vi "RabiMeasurement_IQ2.vi"() -> ()   [LabVIEW 2020]
uses:
  <vilib>/Swabian Instruments/Pulse Streamer/PulseStreamer/PulseStreamer/typedefs/typedef_TriggerStart.ctl
  Host Subvi's/Control 3.ctl
  <vilib>/Swabian Instruments/Pulse Streamer/PulseStreamer/typedefs/typedef_OutputState.ctl
  <vilib>/Swabian Instruments/Pulse Streamer/PulseStreamer/typedefs/typedef_ChannelNumber.ctl
  <vilib>/Swabian Instruments/Pulse Streamer/PulseStreamer/PulsePattern/PulsePattern.lvclass
  C:/Program Files (x86)/National Instruments/LabVIEW 2020/vi.lib/Swabian Instruments/Pulse Streamer/PulseStreamer/Pattern/Pattern.lvclass
  <vilib>/Swabian Instruments/Pulse Streamer/PulseStreamer/Sequence/Sequence.lvclass/Sequence.ctl
  <vilib>/Swabian Instruments/Pulse Streamer/PulseStreamer/AnalogPattern/AnalogPattern.lvclass
  <vilib>/FPGAPlugInAG/USB-7855R/niLvFpga_Open_USB-7855R.vi
  <vilib>/rvi/interface/common/dynamic/niFpgaDynamicAddResources.vi
  <vilib>/rvi/interface/common/niFpgaWaitOnOcc.vi
  <vilib>/Utility/error.llb/Error Cluster From Error Code.vi
  <vilib>/rvi/errors/niLvFpgaAdjustHostInterfaceError.vi
  <vilib>/Swabian Instruments/Pulse Streamer/PulseStreamer/Pattern/Read total duration.vi
  <vilib>/Swabian Instruments/Pulse Streamer/PulseStreamer/PulseStreamer/stream/stream (Sequence).vi
  <vilib>/FPGAPlugInAG/Dynamic/niLvFpga_Close_Dynamic.vi
  <vilib>/rvi/interface/nirviOpenFPGA/nirviOpenFPGA.xnode
  FPGA Bitfiles/EverythingDAQ_FPGATarget2_FPGARabiver2_krdpsiHB5ks.lvbitx
  FPGA_Readout.vi
  <vilib>/rvi/interface/nirviMethod/nirviMethod.xnode
  <vilib>/rvi/interface/nirviCloseFPGA/nirviCloseFPGA.xnode
  <vilib>/Swabian Instruments/Pulse Streamer/PulseStreamer/PulseStreamer/PulseStreamer.lvclass
  <vilib>/Swabian Instruments/Pulse Streamer/PulseStreamer/Sequence/Sequence.lvclass
  <vilib>/FPGAPlugInAG/Dynamic/niLvFpga_ConfigureFifo_Dynamic.vi
  <vilib>/rvi/errors/niLvFpgaMergeErrorWithErrorCode.vi
  <vilib>/FPGAPlugInAG/Dynamic/niLvFpga_WriteFifo_Dynamic.vi
  <vilib>/FPGAPlugInAG/Dynamic/niLvFpga_ReadFifo_Dynamic.vi
  <vilib>/Swabian Instruments/Pulse Streamer/PulseStreamer/PulseStreamer.lvlib
panel:
  out "ESR F2":cluster{"tau array":dbl[], dbl[]}(graph)
  out "ESR F1":cluster{"tau array":dbl[], dbl[]}(graph)
  out "Ave F2":dbl[](array[numeric]) format="%.2f"
  out "Ave F1":dbl[](array[numeric]) format="%.2f"
  out "64bit integer":dbl=22.88
  out "tau array":dbl[](array[numeric])=[2.5, 5.0, 7.5, 10.0, 12.5, 15.0, 17.5, 20.0, 22.5, 25.0, 27.5, 30.0, 32.5, 35.0, 37.5, 40.0, 42.5, 45.0, 47.5, 50.0, 52.5, 55.0, 57.5, 60.0, 62.5, 65.0, 67.5, 70.0, 72.5, 75.0, 77.5, 80.0, 82.5, 85.0, 87.5, 90.0, 92.5, 95.0, 97.5, 100.0, 102.5, 105.0, 107.5, 110.0, 112.5, 115.0, 117.5, 120.0, 122.5, 125.0, 127.5, 130.0, 132.5, 135.0, 137.5, 140.0, 142.5, 145.0, 147.5, 150.0, 152.5, 155.0, 157.5, 160.0, 162.5, 165.0, 167.5, 170.0, 172.5, 175.0, 177.5, 180.0, 182.5, 185.0, 187.5, 190.0, 192.5, 195.0, 197.5, 200.0, 202.5, 205.0, 207.5, 210.0, 212.5, 215.0, 217.5, 220.0, 222.5, 225.0, 227.5, 230.0, 232.5, 235.0, 237.5, 240.0, 242.5, 245.0, 247.5, 250.0, 252.5, 255.0, 257.5, 260.0, 262.5, 265.0, 267.5, 270.0, 272.5, 275.0, 277.5, 280.0, 282.5, 285.0, 287.5, 290.0, 292.5, 295.0, 297.5, 300.0, 302.5, 305.0, 307.5, 310.0, 312.5, 315.0, 317.5, 320.0, 322.5, 325.0, 327.5, 330.0, 332.5, 335.0, 337.5, 340.0, 342.5, 345.0, 347.5, 350.0, 352.5, 355.0, 357.5, 360.0, 362.5, 365.0, 367.5, 370.0, 372.5, 375.0, 377.5, 380.0, 382.5, 385.0, 387.5, 390.0, 392.5, 395.0, 397.5, 400.0, 402.5, 405.0, 407.5, 410.0, 412.5, 415.0, 417.5, 420.0, 422.5, 425.0, 427.5, 430.0, 432.5, 435.0, 437.5, 440.0, 442.5, 445.0, 447.5, 450.0, 452.5, 455.0, 457.5, 460.0, 462.5, 465.0, 467.5, 470.0, 472.5, 475.0, 477.5, 480.0, 482.5, 485.0, 487.5, 490.0, 492.5, 495.0, 497.5, 500.0, 502.5, 505.0, 507.5, 510.0, 512.5, 515.0, 517.5, 520.0, 522.5, 525.0, 527.5, 530.0, 532.5, 535.0, 537.5, 540.0, 542.5, 545.0, 547.5, 550.0, 552.5, 555.0, 557.5, 560.0, 562.5, 565.0, 567.5, 570.0, 572.5, 575.0, 577.5, 580.0, 582.5, 585.0, 587.5, 590.0, 592.5, 595.0, 597.5, 600.0, 602.5, 605.0, 607.5, 610.0, 612.5, 615.0, 617.5, 620.0, 622.5, 625.0, 627.5, 630.0, 632.5, 635.0, 637.5, 640.0, 642.5, 645.0, 647.5, 650.0, 652.5, 655.0, 657.5, 660.0, 662.5, 665.0, 667.5, 670.0, 672.5, 675.0, 677.5, 680.0, 682.5, 685.0, 687.5, 690.0, 692.5, 695.0, 697.5, 700.0, 702.5, 705.0, 707.5, 710.0, 712.5, 715.0, 717.5, 720.0, 722.5, 725.0, 727.5, 730.0, 732.5, 735.0, 737.5, 740.0, 742.5, 745.0, 747.5, 750.0, 752.5, 755.0, 757.5, 760.0, 762.5, 765.0, 767.5, 770.0, 772.5, 775.0, 777.5, 780.0, 782.5, 785.0, 787.5, 790.0, 792.5, 795.0, 797.5, 800.0, 802.5, 805.0, 807.5, 810.0, 812.5, 815.0, 817.5, 820.0, 822.5, 825.0, 827.5, 830.0, 832.5, 835.0, 837.5, 840.0, 842.5, 845.0, 847.5, 850.0, 852.5, 855.0, 857.5, 860.0, 862.5, 865.0, 867.5, 870.0, 872.5, 875.0, 877.5, 880.0, 882.5, 885.0, 887.5, 890.0, 892.5, 895.0, 897.5, 900.0, 902.5, 905.0, 907.5, 910.0, 912.5, 915.0, 917.5, 920.0, 922.5, 925.0, 927.5, 930.0, 932.5, 935.0, 937.5, 940.0, 942.5, 945.0, 947.5, 950.0, 952.5, 955.0, 957.5, 960.0, 962.5, 965.0, 967.5, 970.0, 972.5, 975.0, 977.5, 980.0, 982.5, 985.0, 987.5, 990.0, 992.5, 995.0, 997.5, 1000.0, 1002.5, 1005.0, 1007.5, 1010.0, 1012.5, 1015.0, 1017.5, 1020.0, 1022.5, 1025.0, 1027.5, 1030.0, 1032.5, 1035.0, 1037.5, 1040.0, 1042.5, 1045.0, 1047.5, 1050.0, 1052.5, 1055.0, 1057.5, 1060.0, 1062.5, 1065.0, 1067.5, 1070.0, 1072.5, 1075.0, 1077.5, 1080.0, 1082.5, 1085.0, 1087.5, 1090.0, 1092.5, 1095.0, 1097.5, 1100.0, 1102.5, 1105.0, 1107.5, 1110.0, 1112.5, 1115.0, 1117.5, 1120.0, 1122.5, 1125.0, 1127.5, 1130.0, 1132.5, 1135.0, 1137.5, 1140.0, 1142.5, 1145.0, 1147.5, 1150.0, 1152.5, 1155.0, 1157.5, 1160.0, 1162.5, 1165.0, 1167.5, 1170.0, 1172.5, 1175.0, 1177.5, 1180.0, 1182.5, 1185.0, 1187.5, 1190.0, 1192.5, 1195.0, 1197.5, 1200.0, 1202.5, 1205.0, 1207.5, 1210.0, 1212.5, 1215.0, 1217.5, 1220.0, 1222.5, 1225.0, 1227.5, 1230.0, 1232.5, 1235.0, 1237.5, 1240.0, 1242.5, 1245.0, 1247.5, 1250.0, 1252.5, 1255.0, 1257.5, 1260.0, 1262.5, 1265.0, 1267.5, 1270.0, 1272.5, 1275.0, 1277.5, 1280.0, 1282.5, 1285.0, 1287.5, 1290.0, 1292.5, 1295.0, 1297.5, 1300.0, 1302.5, 1305.0, 1307.5, 1310.0, 1312.5, 1315.0, 1317.5, 1320.0, 1322.5, 1325.0, 1327.5, 1330.0, 1332.5, 1335.0, 1337.5, 1340.0, 1342.5, 1345.0, 1347.5, 1350.0, 1352.5, 1355.0, 1357.5, 1360.0, 1362.5, 1365.0, 1367.5, 1370.0, 1372.5, 1375.0, 1377.5, 1380.0, 1382.5, 1385.0, 1387.5, 1390.0, 1392.5, 1395.0, 1397.5, 1400.0, 1402.5, 1405.0, 1407.5, 1410.0, 1412.5, 1415.0, 1417.5, 1420.0, 1422.5, 1425.0, 1427.5, 1430.0, 1432.5, 1435.0, 1437.5, 1440.0, 1442.5, 1445.0, 1447.5, 1450.0, 1452.5, 1455.0, 1457.5, 1460.0, 1462.5, 1465.0, 1467.5, 1470.0, 1472.5, 1475.0, 1477.5, 1480.0, 1482.5, 1485.0, 1487.5, 1490.0, 1492.5, 1495.0, 1497.5, 1500.0, 1502.5, 1505.0, 1507.5, 1510.0, 1512.5, 1515.0, 1517.5, 1520.0, 1522.5, 1525.0, 1527.5, 1530.0, 1532.5, 1535.0, 1537.5, 1540.0, 1542.5, 1545.0, 1547.5, 1550.0, 1552.5, 1555.0, 1557.5, 1560.0, 1562.5, 1565.0, 1567.5, 1570.0, 1572.5, 1575.0, 1577.5, 1580.0, 1582.5, 1585.0, 1587.5, 1590.0, 1592.5, 1595.0, 1597.5, 1600.0, 1602.5, 1605.0, 1607.5, 1610.0, 1612.5, 1615.0, 1617.5, 1620.0, 1622.5, 1625.0, 1627.5, 1630.0, 1632.5, 1635.0, 1637.5, 1640.0, 1642.5, 1645.0, 1647.5, 1650.0, 1652.5, 1655.0, 1657.5, 1660.0, 1662.5, 1665.0, 1667.5, 1670.0, 1672.5, 1675.0, 1677.5, 1680.0, 1682.5, 1685.0, 1687.5, 1690.0, 1692.5, 1695.0, 1697.5, 1700.0, 1702.5, 1705.0, 1707.5, 1710.0, 1712.5, 1715.0, 1717.5, 1720.0, 1722.5, 1725.0, 1727.5, 1730.0, 1732.5, 1735.0, 1737.5, 1740.0, 1742.5, 1745.0, 1747.5, 1750.0, 1752.5, 1755.0, 1757.5, 1760.0, 1762.5, 1765.0, 1767.5, 1770.0, 1772.5, 1775.0, 1777.5, 1780.0, 1782.5, 1785.0, 1787.5, 1790.0, 1792.5, 1795.0, 1797.5, 1800.0, 1802.5, 1805.0, 1807.5, 1810.0, 1812.5, 1815.0, 1817.5, 1820.0, 1822.5, 1825.0, 1827.5, 1830.0, 1832.5, 1835.0, 1837.5, 1840.0, 1842.5, 1845.0, 1847.5, 1850.0, 1852.5, 1855.0, 1857.5, 1860.0, 1862.5, 1865.0, 1867.5, 1870.0, 1872.5, 1875.0, 1877.5, 1880.0, 1882.5, 1885.0, 1887.5, 1890.0, 1892.5, 1895.0, 1897.5, 1900.0, 1902.5, 1905.0, 1907.5, 1910.0, 1912.5, 1915.0, 1917.5, 1920.0, 1922.5, 1925.0, 1927.5, 1930.0, 1932.5, 1935.0, 1937.5, 1940.0, 1942.5, 1945.0, 1947.5, 1950.0, 1952.5, 1955.0, 1957.5, 1960.0, 1962.5, 1965.0, 1967.5, 1970.0, 1972.5, 1975.0, 1977.5, 1980.0, 1982.5, 1985.0, 1987.5, 1990.0, 1992.5, 1995.0, 1997.5, 2000.0]
  out "t_tot single sequence (ns)":dbl=14300.0
  out "error out 5":errorcluster
  out "Cycle Number 2":i32=70
  in  "Cycle Initialize Tab":enum32{"uWave"}(tab)
  in  "GPIB RF":string="0:27"
  in  "RF Freq (Hz)":dbl=2170000000.0 format="%.5e"
  in  "RF Power (dBm)":dbl=-6.0 format="%.2f"
  in  "uWave Enable":bool=TRUE
  out "RF Freq Set (GHz)":dbl=2.17 format="%#_10f"
  in  "Delay (ns)":T1=760
  in  "start":T2
  in  "ip":string="169.254.8.2"
  in  "?":enum32{"Confocal"}(tab)
  in  "x":i16=77
  in  "y":i16=76
  in  "Scan Area":i16=1
  in  "Scale (1-30)":i16=4
  in  "Sample per Axis":i16=151
  in  "?":enum32{"Rabi"}(tab)
  in  "Wait Time (ns)":u32=2300
  in  "Initialization time (ns)":u32=5240
  in  "Readout (ns)":u32=6000
  in  "Number of points":u32=800
  in  "Pulse Num":u32=500
  in  "Experiment Repeat":i32=500
  out "Experiment number":i32=95
  out "n_runs":i64=500
  in  "tau start (ns)":dbl=2.5
  in  "tau step (ns)":dbl=2.5
  out "error out 4":errorcluster
  out "Digital plot":cluster{"CumTime":i64[], dbl[]}[](graph)
  out "error out 3":errorcluster
  out "Sequence duration [ms]":dbl=11440.0 format="%.2f"
  out "N_array":i32[](array[numeric])=[0, 1, 2, 3, 4, 5, 6, 7, 8, 9, 10, 11, 12, 13, 14, 15, 16, 17, 18, 19, 20, 21, 22, 23, 24, 25, 26, 27, 28, 29, 30, 31, 32, 33, 34, 35, 36, 37, 38, 39, 40, 41, 42, 43, 44, 45, 46, 47, 48, 49, 50, 51, 52, 53, 54, 55, 56, 57, 58, 59, 60, 61, 62, 63, 64, 65, 66, 67, 68, 69, 70, 71, 72, 73, 74, 75, 76, 77, 78, 79, 80, 81, 82, 83, 84, 85, 86, 87, 88, 89, 90, 91, 92, 93, 94, 95]
  out "CountAverage":dbl[](array[numeric])=[2.2072775, 2.1462875, 2.1518225, 2.13079, 2.1088175, 2.0855425, 2.092535, 2.095995, 2.059395, 2.043535, 2.0711575, 2.0722175, 2.0613325, 2.0553225, 2.05686, 2.06965, 2.0412975, 2.0224125, 2.03104, 2.0491125, 2.0315925, 2.05474, 2.070495, 2.0499125, 2.00775, 2.0107775, 1.981505, 1.9941775, 1.9933125, 1.97172, 1.9845575, 1.998325, 1.9735575, 1.9803825, 2.006115, 1.999575, 2.010875, 1.9825875, 1.9527725, 1.9487225, 1.9575375, 1.94913, 1.9602425, 1.97378, 1.9248975, 1.95134, 1.95578, 1.93173, 1.96891, 1.9429025, 1.94519, 1.9535725, 1.982075, 1.9884975, 2.0101, 2.0035625, 1.9885975, 1.9950825, 1.9905625, 2.0166725, 2.0082125, 1.979385, 1.9926625, 1.99645, 1.96617, 1.994985, 2.02208, 2.02243, 1.98502, 2.030615, 1.95893, 1.950755, 1.954205, 1.9540825, 2.001115, 2.0058825, 1.98758, 2.0253575, 2.0277525, 2.018475, 2.0500375, 1.996235, 2.002115, 1.98259, 1.9926, 2.0195225, 2.03915, 2.005845, 1.9993925, 1.97835, 1.97021, 1.971995, 1.9831425, 2.0152025, 2.005475]
  out "Averaged ESR":dbl[](array[numeric])=[1.017870567091982, 1.0428926603215876, 1.0764184990280088, 1.08249192001354, 1.09429499579298, 1.1037168082128996, 1.1050716542744574, 1.1014298057989265, 1.089578613265814, 1.0709781534452711, 1.061324574848865, 1.0399698584374584, 1.0274961657701196, 1.0323259829375757, 1.049009998093537, 1.06086353915061, 1.073642946086008, 1.0916880804324838, 1.1136897270610668, 1.1028359205101759, 1.1019091471026512, 1.0875769519321419, 1.0844743820788172, 1.0759806167827617, 1.0442674590752932, 1.048090882105439, 1.0495594176031688, 1.0518328239293575, 1.0687563191014522, 1.0818212468587356, 1.0882605899283622, 1.096100309473077, 1.1037350318350123, 1.1156983902933313, 1.1020839762563372, 1.0905140527288388, 1.0815812888771692, 1.0642144974277141, 1.0579398581706974, 1.0586754609636846, 1.0624506346078841, 1.0634495683486118, 1.0700074839543063, 1.07995537502229, 1.0894526493826528, 1.1013206815502923, 1.1003407028071455, 1.1022423549057012, 1.0954878362287324, 1.088062027708647, 1.0833266346542303, 1.076664423393035, 1.078449296773364, 1.0705152899378316, 1.0706985926619503, 1.0773806630088303, 1.0862648694729151, 1.0947271213098375, 1.098040473863476, 1.1057727933875288, 1.1001579636399577, 1.100441019528767, 1.0887476609105367, 1.0937902660037309, 1.0787961808148738, 1.0767806248990635, 1.0723241131589933, 1.0745023953966337, 1.0772759452030733, 1.0802973083495904, 1.089253522438231, 1.095749559409236, 1.0918005448710129, 1.1055463304557207, 1.0999171683721327, 1.1008361418047856, 1.092833534540528, 1.0890529342944788, 1.095166497145744, 1.0889157153776328, 1.085628303208282, 1.0781862682944452, 1.0821695429125877, 1.0925768644288618, 1.098383847187047, 1.0944772252952568, 1.1023227543449177, 1.097807910096037, 1.1009879373329856, 1.0877833673466615, 1.0861943902564453, 1.0938514691759695, 1.0973681152773327, 1.0896493347316616, 1.0995933627888295, 1.088455035810942, 1.098379320211397, 1.0932950865725335, 1.0961741121162156, 1.113305342500775, 1.101220239196636, 1.0974704662525034, 1.0940260344564623, 1.099352223526442, 1.0946502698139342, 1.0946253871244664, 1.097434654594297, 1.0925623295543303, 1.0919700367152774, 1.0895337606212658, 1.0972227873890035, 1.094692169210638, 1.0987845450816978, 1.0959354792682467, 1.102933736999957, 1.10373081009968, 1.1010789380405153, 1.0911602135159661, 1.1051350650124456, 1.0882875705674595, 1.0935795187132247, 1.0961128747578008, 1.0940564931044212, 1.0907245409372075, 1.086972927097673, 1.101921669694619, 1.1045386541333555, 1.0968130982139743, 1.099319216745386, 1.0980869935384356, 1.1002204797692952, 1.0948595192314083, 1.090853656099697, 1.0899171335680933, 1.1066240994796002, 1.104192116433813, 1.099298327935454, 1.1051796023445397, 1.1003176925572662, 1.1003755408993299, 1.105582846608761, 1.106507276056704, 1.1022924612455625, 1.1080644274971405, 1.0952665177369774, 1.1075785062314032, 1.112163765039852, 1.1090146896467583, 1.1072604739666427, 1.0898761474764147, 1.0984143910384845, 1.1107980671802806, 1.109894367537097, 1.0954476327698346, 1.1014993452209336, 1.104524478619451, 1.0990222514128662, 1.1062364223321395, 1.117382720986981, 1.1009953112710726, 1.0988904397545864, 1.1095039144640335, 1.1014771334737596, 1.104214998620112, 1.1034419330780372, 1.1036389406502143, 1.1040262882497887, 1.1006839694366446, 1.1134296632704657, 1.1162085672629536, 1.1008701821707778, 1.1056496739630912, 1.1080773760250575, 1.10565621829497, 1.0936325898364008, 1.1113592863916006, 1.109594455045102, 1.1041919238247428, 1.1091828926384746, 1.1052749226278205, 1.100626534503294, 1.1145255572300725, 1.105475777135918, 1.1161846296087823, 1.1059302766646626, 1.0984978688159608, 1.1040162611639632, 1.1067951207834936, 1.106398199393047, 1.1015433879679135, 1.1092495655208994, 1.1052989922635286, 1.1213348020476828, 1.11442191453326, 1.1126210753135222, 1.1062278750292944, 1.1129922330823754, 1.1112575296397664, 1.106995206046034, 1.105772584152529, 1.1046626229036116, 1.105620739100793, 1.1030560137251477, 1.0987158149207024, 1.1098403421070224, 1.1024548032168695, 1.1174986138576837, 1.1134012388413053, 1.1186445977943822, 1.1107554917486824, 1.1137660120736623, 1.1107915302247544, 1.100391880715458, 1.1088381178257134, 1.1073906612240598, 1.1111821517005023, 1.111279669108648, 1.117205324051906, 1.111138122017584, 1.107469828805801, 1.1107833057587215, 1.106007992494114, 1.1107163808717235, 1.108369276034106, 1.1119579127443364, 1.1191663643085161, 1.1145945822584509, 1.1082270728510075, 1.1021618478400625, 1.1128436007246514, 1.1156632372941158, 1.1117635252190883, 1.1108565390750174, 1.1143026054777658, 1.1135125479380992, 1.1048708380999308, 1.110978437212152, 1.107832934669327, 1.1083019799037073, 1.1171085710654212, 1.109674255062311, 1.1172280795952831, 1.0966895456362442, 1.1114427385391759, 1.112558678819698, 1.1159257515149266, 1.1170847002606754, 1.1091079392837468, 1.1252746176368875, 1.1164868747994192, 1.1115257272765922, 1.112492715526884, 1.1131721874913165, 1.106415955928393, 1.1127515047130214, 1.121777404855146, 1.1113917400138986, 1.1065610049641, 1.112886183137908, 1.120325908446153, 1.111955487046645, 1.1151325838576336, 1.0968828462071702, 1.1108731419559708, 1.1052816763772486, 1.1072028238831386, 1.11923405291813, 1.117043314690874, 1.1155127042804995, 1.1161604913932, 1.1090132956955054, 1.1185718347159035, 1.110163718540335, 1.1094259675763776, 1.1208428601364433, 1.113265417625146, 1.114188464397012, 1.1041508706085694, 1.1157251980105294, 1.127667927988856, 1.125019388249312, 1.114052470720931, 1.1054909705514124, 1.117017337834489, 1.1093217690333856, 1.1131590904758164, 1.1165869621422975, 1.118603082160916, 1.119290885713883, 1.122997947042949, 1.1217670088955027, 1.1238244918431606, 1.1153859289299557, 1.1180327605088434, 1.111799822079564, 1.125498317085623, 1.1157273631724003, 1.1171976776520487, 1.108180640821213, 1.1269659320725054, 1.1076175099737944, 1.1178968399028157, 1.1181458276217189, 1.1159379955502584, 1.1104726176802293, 1.1207848568303298, 1.1155542613176883, 1.122145322667982, 1.1222585006478654, 1.1174016036964423, 1.1176550500904248, 1.1243703040970456, 1.1159524441907427, 1.1214840172417146, 1.116292485364949, 1.1160786722521903, 1.1188233095548725, 1.1160594543237685, 1.1152657523041858, 1.1195265583309715, 1.1158828916271493, 1.1243780078300036, 1.1209660018460017, 1.1195362387898076, 1.1198173858626708, 1.1183999021996651, 1.1224124216220939, 1.112000997216563, 1.1240473046136088, 1.1218271745243493, 1.1324092229410991, 1.1235014370498202, 1.1183973471070325, 1.1242992481028977, 1.1115671103971074, 1.1146129171862327, 1.1041438428142174, 1.118209285965627, 1.1209125677876899, 1.116192905756716, 1.1242474075797333, 1.115426073604158, 1.117683871762317, 1.1208561818335452, 1.1169558107602149, 1.1270683431645778, 1.1204730512986776, 1.1150402816372227, 1.1209408034389028, 1.11824649079262, 1.1223299357092964, 1.1181149372744197, 1.1274976794403853, 1.1223018952815542, 1.12895534812574, 1.1265498885641079, 1.12735612050998, 1.129742695850777, 1.1160852670845944, 1.1162574861324048, 1.1222591386084062, 1.125229525973104, 1.1157566201244884, 1.1207123280773603, 1.1145647004665675, 1.1210114918086267, 1.1176168918049203, 1.1269815176426483, 1.1235793352163512, 1.1268882863132637, 1.1173733155272814, 1.1325302764619436, 1.1225230426410628, 1.1141307565157381, 1.1293595976168223, 1.1287265502460078, 1.122215914161613, 1.1263042025389576, 1.1213518705793615, 1.122534695610121, 1.1212848902002543, 1.1236269050663472, 1.1223110261430218, 1.1141658382693735, 1.1270678768039786, 1.1236500582586075, 1.1214985254815095, 1.1306999083034452, 1.122796553412026, 1.1254558573041624, 1.1207807940227021, 1.1294424950373962, 1.134143206526851, 1.1255481494610171, 1.1270780880161722, 1.1241813431432839, 1.122413221191102, 1.1214597630957202, 1.1173917280611008, 1.1280768573501714, 1.1338056271405481, 1.1202075594212675, 1.1278318833938057, 1.1323799830183578, 1.1267732442724232, 1.1269699824451824, 1.1303804382519782, 1.1218198297824533, 1.1232426214056597, 1.1234647259277108, 1.1192548412415468, 1.1194774190617316, 1.1234105721000718, 1.1190794875575931, 1.1254410892590854, 1.1226844359172394, 1.1191686645401684, 1.127482697490476, 1.1299411893890805, 1.1220893059031614, 1.119214739194092, 1.1229301672480712, 1.1359371936969012, 1.122894017158999, 1.115512241425835, 1.122681522992113, 1.122654808493137, 1.1193516177925849, 1.126640257005834, 1.1252516181167556, 1.1192775442772362, 1.1214721961303855, 1.1269430509253915, 1.1269493106173074, 1.1228485289694627, 1.1205968851106325, 1.1313313737541615, 1.1257948065155983, 1.1260294831969244, 1.1333863505745625, 1.1348761316788354, 1.121377533937546, 1.1215368954556886, 1.1216920334212717, 1.1171356177618341, 1.1289950580764188, 1.1302556712087384, 1.1198489636019553, 1.132767811128869, 1.1266107519168016, 1.1289786041054588, 1.1270041694564048, 1.1198646493440356, 1.1164296128853253, 1.1184833921512385, 1.1285583470465177, 1.1288891261981928, 1.1213252926737172, 1.1311641903602372, 1.1358343135057054, 1.123185311806359, 1.1316403984000385, 1.1277173525169113, 1.1246851026658191, 1.1489188870953129, 1.1213776761706984, 1.126454365986109, 1.129379383353563, 1.1326305493724642, 1.1260299759908172, 1.1284717768296124, 1.124683449514201, 1.129492979194873, 1.1332389844719708, 1.1346100624609043, 1.1302245740579817, 1.1208098447083643, 1.121062914306376, 1.1336996946105724, 1.129989026110717, 1.1385121944696786, 1.1387939494498163, 1.1361036047089081, 1.1315831258458675, 1.1249482657215217, 1.140939940864156, 1.1244942412033658, 1.1268625836214707, 1.1198544446059677, 1.1195130292511157, 1.128745658774659, 1.1197909586282588, 1.1293450177738118, 1.1240123670586861, 1.1364420944442386, 1.1294726402361845, 1.1382326066000212, 1.1206736483332902, 1.1303310200501433, 1.1344319764752102, 1.1229958779702038, 1.1281101893631422, 1.134418740863535, 1.1235822411589944, 1.1305734549470545, 1.1237239329680047, 1.127987506092654, 1.1236047664643987, 1.1315210451691822, 1.1342939418124094, 1.1333263387028139, 1.126377472422558, 1.127660770303706, 1.1301314550774404, 1.1230503737511595, 1.1250667584725844, 1.1312853803668195, 1.1314963531556166, 1.1319076228929146, 1.1234297316738115, 1.1232159018241141, 1.1213863310402332, 1.1330437995742415, 1.125385723163931, 1.1340479059652335, 1.1421450999195475, 1.1397426466624196, 1.1316064331995206, 1.1297916859225872, 1.1354144860328363, 1.136023056921058, 1.132351000373656, 1.1239134293359985, 1.1307159054669231, 1.1243527172955214, 1.138621487734734, 1.1240956128498698, 1.1207479991237073, 1.1338378644026976, 1.1338742459275484, 1.1305469914586572, 1.1254126672670035, 1.1273875871978445, 1.1317119124396593, 1.1369676440202887, 1.1314151908507226, 1.1302356417590398, 1.113156316359339, 1.1338583366506407, 1.1337549337030488, 1.1337932105887751, 1.1326882578808375, 1.1385578711499684, 1.125576870406502, 1.1225225279410291, 1.1317744964193017, 1.1219050927198981, 1.1251569936048238, 1.1326536139829566, 1.1275566401784909, 1.1297569229358313, 1.129862201324187, 1.124118856741387, 1.1315753136253772, 1.1284838436749562, 1.1290830020821105, 1.1224286157692762, 1.1262046491066684, 1.1313974298463507, 1.1365711521763828, 1.1241388774181382, 1.1345599158203457, 1.1320225507589132, 1.1283706378817295, 1.1252211603716062, 1.138282978252128, 1.1308128604600702, 1.129231815390267, 1.1327363850546435, 1.1271993786956445, 1.1404355025443793, 1.1281413710787662, 1.1284024558970245, 1.133685363253103, 1.131591236954282, 1.1406814477818061, 1.1365441631670428, 1.125847976347756, 1.1328581700881377, 1.1310800012589288, 1.1366196381689113, 1.1280658765395304, 1.1332264299966262, 1.1304109490182934, 1.132535892926528, 1.1301541978517515, 1.1311294932632443, 1.131109822660871, 1.1241702928321666, 1.1236375478731322, 1.1257060368177922, 1.130639171298709, 1.1349415434844579, 1.1478914111199454, 1.1286488787079925, 1.1305522316217547, 1.141308302506417, 1.135669679535242, 1.1251414585283825, 1.1334191696777076, 1.1326844175179327, 1.1354064498355063, 1.1309995009972904, 1.1446147623229164, 1.1171683258219194, 1.1336885766414995, 1.1287433400630595, 1.1313728969378958, 1.1381222453839939, 1.1308686743171255, 1.14527778393921, 1.1287019075870957, 1.1187262461040786, 1.120329101539357, 1.1359609279480767, 1.1325065530525351, 1.13832581255246, 1.1353034414412362, 1.1426406165520944, 1.1373579270587468, 1.1302655900093561, 1.1389014914340951, 1.143931651063482, 1.1297139801384206, 1.128872058158146, 1.125538993667513, 1.1396843555879195, 1.1319961336156976, 1.1241665001500885, 1.1331447326523847, 1.1270711534746813, 1.1339766507241806, 1.1313552155139543, 1.131923494696269, 1.133713208863953, 1.1311043781846715, 1.137220900182611, 1.1247900947402854, 1.1373274380942666, 1.1384604517257901, 1.13746478720897, 1.1289327975596795, 1.1413214641791471, 1.1257688518435236, 1.1410842959494842, 1.1316359756372707, 1.1363876950639915, 1.1370497125710388, 1.142822491230249, 1.1350073449247742, 1.1249265270029862, 1.1369947487049261, 1.1261831627736012, 1.130905110426474, 1.1383158515457605, 1.1369849861682004, 1.1325204894650371, 1.1309130590498722, 1.1251576981026314, 1.133190148560051, 1.1385501477376463, 1.1308727614375844, 1.1340737433096648, 1.1269706792076597, 1.1320709423684914, 1.1339516324670158, 1.1470304047023454, 1.1449383393860684, 1.136093733212451, 1.1370435455791412, 1.1379704057751572, 1.1367747812181677, 1.1388017915960975, 1.1299824376992134, 1.1303433567675798, 1.122845097958489, 1.1361919544398191, 1.135183549829578, 1.1280804942569518, 1.131941502025668, 1.136980554771434, 1.1404810574511153, 1.1350873904823944, 1.1314576924428175, 1.127720945589, 1.1457972884773437, 1.1339509316120857, 1.1288714659519623, 1.129025444261436, 1.1347252645728116, 1.127048523684636, 1.1377569666587408, 1.1364972600327, 1.1286657041750106, 1.1265519810294022, 1.1433104502210911, 1.136847235197547, 1.1270108693214904, 1.1418492577465624, 1.130973249736025, 1.133005722747554, 1.1299941097590815, 1.1302650303886679, 1.137273036226643, 1.1451237531270146, 1.1326751309039664, 1.1294341413389932, 1.1346959126105762, 1.135603784564775, 1.136326971353465, 1.135217672302347, 1.1321252889264852, 1.131185230055024, 1.1270786047741617, 1.1322835621377718, 1.134308457905249, 1.1383964871741532, 1.1409670200352167, 1.1425944598419815, 1.1257998725902563, 1.1358828900529776, 1.1314930034650579, 1.1419359310342247, 1.1320140266233798, 1.1272241338433864, 1.1450985134963882, 1.1391845878613314, 1.137886980973463, 1.1461572113907659, 1.1412976300369604, 1.1321946222419996, 1.1354188355391885, 1.130733406546916, 1.138804076769946, 1.1332926964998102, 1.1352202305235357, 1.1476563442612666, 1.1273956171359665, 1.1385466038066507, 1.145954275421024, 1.1280223539434222, 1.1348840010810184, 1.1493421384567841, 1.1341140536354464, 1.1293148751132422, 1.142676625767849, 1.1424198941878665, 1.131572893783053, 1.1282676893521884, 1.1381627679227357, 1.1308610089277378, 1.131284159607972, 1.1318539286805007, 1.1357926078703677, 1.1361172850773913, 1.1393549176859867, 1.146707791746724, 1.1396525953233352, 1.1417747625988734, 1.1452429297343047, 1.130271620049661, 1.1317075306351825, 1.1331998086671642, 1.1419446607720263, 1.134491962629883, 1.139594266978447, 1.1433427269412335, 1.1343674572867815, 1.1291268386803468, 1.1348539789874885, 1.1392296684413437, 1.1314778005332473, 1.1384866944880645, 1.1393698972706916, 1.1436734829042945, 1.1393695568663702, 1.131669082749806, 1.1394655856344118, 1.1297977711820328, 1.1450732771866803, 1.1305843914326033, 1.1325734898833544, 1.1385865919493063, 1.1336892060704917, 1.136953405091708, 1.136019336506689, 1.1389285870307104, 1.1324377189751336, 1.138519289522576, 1.1313850424791982]
  out "Empty Elements Remaining 2":u32=1712128
  out "Rabi plot":cluster{"tau array":dbl[], dbl[]}(graph)
  out "Average Counts":cluster{"N_array":i32[], "CountAverage":dbl[]}(graph)={"N_array"=[0, 1, 2, 3, 4, 5, 6, 7, 8, 9, 10, 11, 12, 13, 14, 15, 16, 17, 18, 19, 20, 21, 22, 23, 24, 25, 26, 27, 28, 29, 30, 31, 32, 33, 34, 35, 36, 37, 38, 39, 40, 41, 42, 43, 44, 45, 46, 47, 48, 49, 50, 51, 52, 53, 54, 55, 56, 57, 58, 59, 60, 61, 62, 63, 64, 65, 66, 67, 68, 69, 70, 71, 72, 73, 74, 75, 76, 77, 78, 79, 80, 81, 82, 83, 84, 85, 86, 87, 88, 89, 90, 91, 92, 93, 94], "CountAverage"=[2.2072775, 2.1462875, 2.1518225, 2.13079, 2.1088175, 2.0855425, 2.092535, 2.095995, 2.059395, 2.043535, 2.0711575, 2.0722175, 2.0613325, 2.0553225, 2.05686, 2.06965, 2.0412975, 2.0224125, 2.03104, 2.0491125, 2.0315925, 2.05474, 2.070495, 2.0499125, 2.00775, 2.0107775, 1.981505, 1.9941775, 1.9933125, 1.97172, 1.9845575, 1.998325, 1.9735575, 1.9803825, 2.006115, 1.999575, 2.010875, 1.9825875, 1.9527725, 1.9487225, 1.9575375, 1.94913, 1.9602425, 1.97378, 1.9248975, 1.95134, 1.95578, 1.93173, 1.96891, 1.9429025, 1.94519, 1.9535725, 1.982075, 1.9884975, 2.0101, 2.0035625, 1.9885975, 1.9950825, 1.9905625, 2.0166725, 2.0082125, 1.979385, 1.9926625, 1.99645, 1.96617, 1.994985, 2.02208, 2.02243, 1.98502, 2.030615, 1.95893, 1.950755, 1.954205, 1.9540825, 2.001115, 2.0058825, 1.98758, 2.0253575, 2.0277525, 2.018475, 2.0500375, 1.996235, 2.002115, 1.98259, 1.9926, 2.0195225, 2.03915, 2.005845, 1.9993925, 1.97835, 1.97021, 1.971995, 1.9831425, 2.0152025, 2.005475]}
  in  "Save Data":bool
  out "Elements Remaining":u32
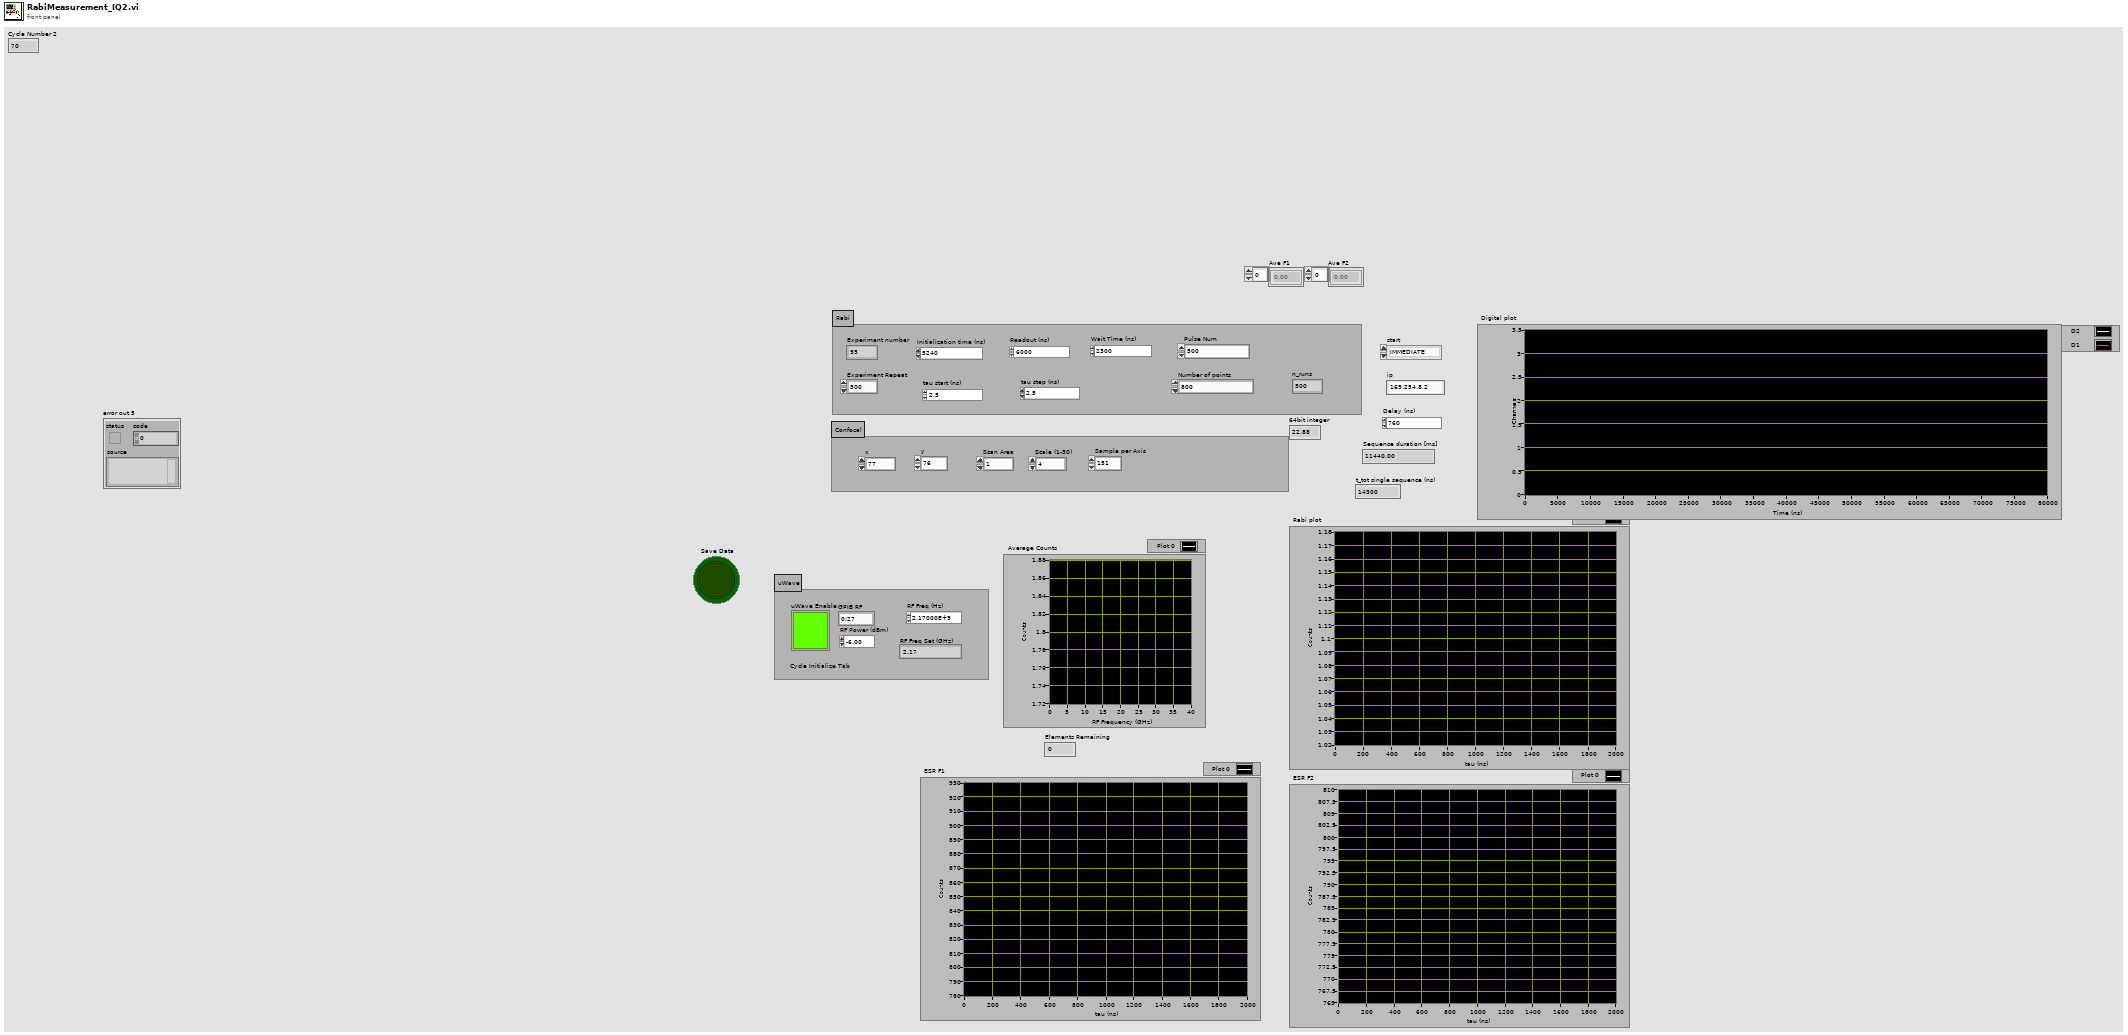
[diagram p1: front panel]
types:
  T1 = typedef "Control 3.ctl" = u32
  T2 = typedef "PulseStreamer.lvlib/PulseStreamer.lvclass/typedef_TriggerStart.ctl" = enum16{"IMMEDIATE", "SOFTWARE", "HW_RISING", "HW_FALLING", "HW_RISING_AND_FALLING"}
  T3 = typedef "PulseStreamer.lvlib/typedef_ChannelNumber.ctl" = i16
  T4 = typedef "PulseStreamer.lvlib/typedef_OutputState.ctl" = cluster{"channels":T3[], "a0":dbl, "a1":dbl}
  T5 = typedef "PulseStreamer.lvlib/typedef_DeviceInfo.ctl" = cluster{"ip":string, "serial":string, "hostname":string, "model":string, "firmware":string, "fpgaid":string, "hardware":string}
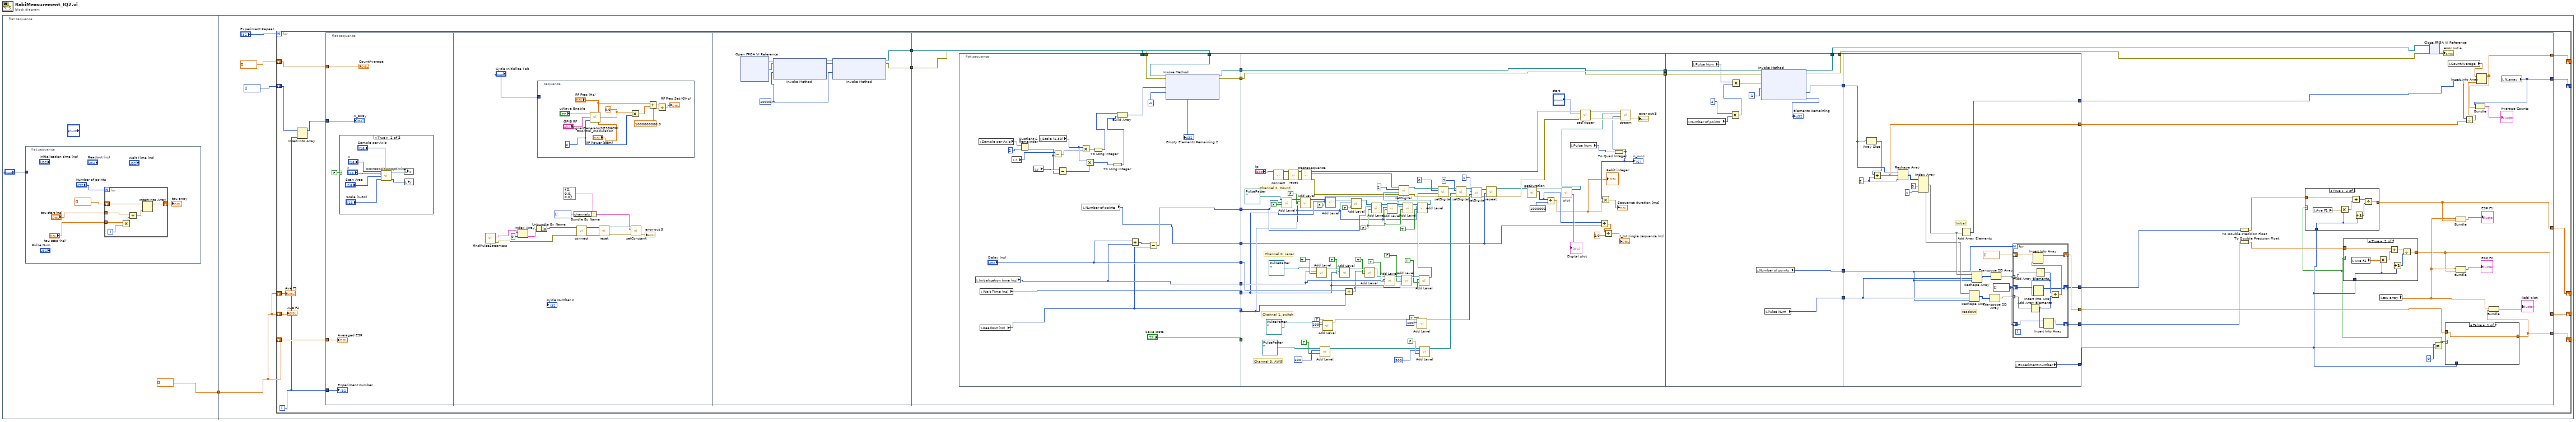
[diagram p0: block diagram]
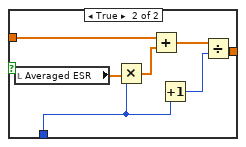
[diagram p5: hidden frame]
diagram:
  n1 = flat-sequence {
    tunnel: [dbl[] [] ("Averaged ESR")] -> w1
    tunnel: w1 -> [w16]
    frame #0 {
      n2 = flat-sequence {
        tunnel: "?" -> [_]
        frame #0 {
          n3 = for {
            N: "Number of points" -> [_]
            tunnel: "tau step (ns)" -> [w14]
            tunnel: "tau start (ns)" -> [w12]
            shift-right: [w9] -> w5
            shift-left: dbl[] [] -> [w10]
            i -> [w15]
            n4 = Multiply(x=w14, y=w15) -> (x*y=w13:dbl)
            n5 = Add(x=w12, y=w13) -> (x+y=w11:dbl)
            n6 = Insert Into Array(array=w10, new element=w11) -> (w9:dbl[])  [unwired: 1 in]
          }
          "tau array" <- w5
        }
      }
    }
    frame #1 {
      n7 = for {
        N: "Experiment Repeat" -> [_]
        shift-right: [w33] -> _
        shift-left: w16 -> [w27]
        shift-right: [w32] -> _
        shift-left: dbl[] [] -> [w25]
        shift-right: [w30] -> _
        shift-left: i32[] [] ("N_array") -> [w31]
        shift-right: [w20] -> _
        shift-left: w16 -> [w21]
        shift-right: [w23] -> _
        shift-left: w16 -> [w22]
        i -> [w24]
        n8 = Insert Into Array(array=w31, new element=w24) -> (w26:i32[])  [unwired: 1 in]
        n9 = flat-sequence {
          tunnel: w27 -> [w38]
          tunnel: w26 -> [w37]
          tunnel: w25 -> [w36]
          tunnel: w24 -> [w35]
          tunnel: [w72] -> w29
          tunnel: [w71] -> w28
          tunnel: [w116] -> w33
          tunnel: [w114] -> w32
          tunnel: [w113] -> w30
          tunnel: w29 -> [w110]
          tunnel: w28 -> [w109]
          tunnel: [w80] -> w23
          tunnel: [w81] -> w20
          frame #0 {
            n10 = case shown="True" FALSE {
              frame False {
              }
              frame True {
                n11 = call "ODMRPositionOptimize.vi"("x"="x", "y"="y", "Scan Area"="Scan Area", "Scale (1-30)"="Scale (1-30)", "Sample per Axis"="Sample per Axis") -> ("Optimized X"=w41:i32, "Optimized Y"=w40:i32)  [unwired: 1 in]
                n12 = local write "x"(w41) -> ()
                n13 = local write "y"(w40) -> ()
              }
            }
            "Averaged ESR" <- w38
            "N_array" <- w37
            "CountAverage" <- w36
            "Experiment number" <- w35
          }
          frame #1 {
            n14 = call <vilib>:"findPulseStreamers.vi"() -> ("error out"=w47:errorcluster, "Descriptions"=w48:T5[])  [unwired: 10 in]
            n15 = Index Array(array=w48, index=0) -> (element=w57:T5)
            n16 = Unbundle By Name(w57) -> ("ip"=w56:string)
            n17 = stacked-sequence {
              tunnel: "Cycle Initialize Tab" -> [_]
              frame #0 {
                w67 = 0.0 ("RF Freq Step (Hz)")
                w63 = 0 ("y")
                n18 = call "SignalGeneratorSG386GPIBControl_modulation.vi"("RF Power (dBm)"="RF Power (dBm)", "RF Freq Step (Hz)"=w67, "RF Freq (Hz)"="RF Freq (Hz)", "Current loop"=w63, "GPIB RF"="GPIB RF", "uWave Enable"="uWave Enable") -> ()
                n19 = Multiply(x=w67, y=w63) -> (x*y=w65:dbl)
                n20 = Add(x="RF Freq (Hz)", y=w65) -> (x+y=w62:dbl)
                n21 = Divide(x=w62, y=1000000000.0) -> (x/y=→"RF Freq Set (GHz)":dbl)
              }
            }
            n22 = Bundle By Name(cluster=T4 {"channels"=[], "a0"=0.0, "a1"=0.0} ("OutputState"), "channels"=T3[] []) -> (w50:T4)
            n23 = call <vilib>:"connect.vi"("error in (no error)"=w47, "ip"=w56) -> ("error out"=w54:errorcluster, "Pulse Streamer out"=w55:refnum<class "PulseStreamer.lvclass">)  [unwired: 8 in]
            n24 = call <vilib>:"reset.vi"("error in (no error)"=w54, "Pulse Streamer in"=w55) -> ("error out"=w51:errorcluster, "Pulse Streamer out"=w52:refnum<class "PulseStreamer.lvclass">)  [unwired: 8 in]
            n25 = call-dynamic "setConstant.vi"("error in (no error)"=w51, "outputState"=w50, "Pulse Streamer in"=w52) -> ("error out"=→"error out 5":errorcluster)  [unwired: 7 in, 1 out]
          }
          frame #2 {
            w76 = u32 10000 ("Requested Depth")
            n26 = xnode "Open FPGA VI Reference"() -> ("FPGA VI Reference Out"=w73:refnum<k20>, "error out"=w70:errorcluster)  [unwired: 2 in]
            n27 = xnode "Invoke Method"("FPGA VI Reference In"=w73, "error in"=w70, "Requested Depth"=w76) -> ("FPGA VI Reference Out"=w74:refnum<k20>, "error out"=w75:errorcluster)  [unwired: 1 out]
            n28 = xnode "Invoke Method"("FPGA VI Reference In"=w74, "error in"=w75, "Requested Depth"=w76) -> ("FPGA VI Reference Out"=w72:refnum<k20>, "error out"=w71:errorcluster)  [unwired: 1 out]
          }
          frame #3 {
            n29 = flat-sequence {
              tunnel: ["Save Data"] -> w104
              tunnel: [w137] -> w103
              tunnel: [w139] -> w102
              tunnel: [w135] -> w101
              tunnel: w110 -> [w145]
              tunnel: w110 -> [_]
              tunnel: w109 -> [w144]
              tunnel: [w142] -> w100
              tunnel: [w141] -> w99
              tunnel: ["Delay (ns)"] -> w98
              tunnel: [w136] -> w97
              tunnel: [w134] -> w93
              tunnel: w104 -> [_]
              tunnel: [w223] -> w96
              tunnel: [w222] -> w95
              tunnel: w103 -> [w189]
              tunnel: w102 -> [w195]
              tunnel: w101 -> [w190]
              tunnel: w100 -> [w223]
              tunnel: w99 -> [w222]
              tunnel: w98 -> [w218]
              tunnel: w97 -> [w202]
              tunnel: w93 -> [w181]
              tunnel: [w261] -> w94
              tunnel: w96 -> [w260]
              tunnel: w95 -> [w259]
              tunnel: [w258] -> w107
              tunnel: [w257] -> w106
              tunnel: [w254] -> w91
              tunnel: [w253] -> w90
              tunnel: w94 -> [w279]
              tunnel: [w285] -> w89
              tunnel: [w280] -> w92
              tunnel: w91 -> [w270]
              tunnel: w90 -> [w271]
              tunnel: [w269] -> w88
              tunnel: [w268] -> w85
              tunnel: [w265] -> w87
              tunnel: [w264] -> w84
              frame #0 {
                n30 = local read "Initialization time (ns)"() -> (w139:u32)
                n31 = local read "Sample per Axis"() -> (w158:i16)
                n32 = local read "Wait Time (ns)"() -> (w135:u32)
                n33 = local read "Readout (ns)"() -> (w137:u32)
                n34 = local read "x"() -> (w157:i16)
                n35 = Quotient & Remainder(x=w158, y=i16 2) -> (floor(x/y)=w155:i16)  [unwired: 1 out]
                n36 = local read "y"() -> (w156:i16)
                n37 = local read "Scale (1-30)"() -> (w153:i16)
                n38 = Subtract(x=w157, y=w155) -> (x-y=w148:i16)
                n39 = Subtract(x=w156, y=w155) -> (x-y=w154:i16)
                n40 = Multiply(x=w153, y=w148) -> (x*y=w152:i16)
                n41 = local read "Number of points"() -> (w134:u32)
                n42 = Multiply(x=w153, y=w154) -> (x*y=w150:i16)
                n43 = To Long Integer(number=w152) -> (32bit integer=w151:i32)
                n44 = To Long Integer(number=w150) -> (32bit integer=w149:i32)
                n45 = Build Array(w151, w149) -> (w143:i32[])
                n46 = Add(x="Delay (ns)", y=w139) -> (x+y=w138:T1)
                n47 = Subtract(x=w138, y=w137) -> (x-y=w136:T1)
                n48 = xnode "Invoke Method"("FPGA VI Reference In"=w145, "error in"=w144, "Data"=w143, "Timeout (ms)"=-1) -> ("FPGA VI Reference Out"=w142:refnum<k20>, "error out"=w141:errorcluster, "Empty Elements Remaining"=→"Empty Elements Remaining 2":u32)
              }
              frame #1 {
                w203 = FALSE ("Level")
                # "Channel 3, AWG"
                # "Channel 1, switch"
                # "Channel 0, Laser"
                # "Channel 2, Count"
                n49 = call <vilib>:"connect.vi"("ip"="ip") -> ("error out"=w236:errorcluster, "Pulse Streamer out"=w237:refnum<class "PulseStreamer.lvclass">)  [unwired: 9 in]
                n50 = call <vilib>:"Add Level.vi"("Level"=FALSE, "Duration"=w202, "Digital Sequence in"=refnum<class "PulsePattern.lvclass"> refnum) -> ("Digital Sequence out"=w217:refnum<class "PulsePattern.lvclass">)  [unwired: 8 in]
                n51 = call <vilib>:"reset.vi"("error in (no error)"=w236, "Pulse Streamer in"=w237) -> ("error out"=w239:errorcluster, "Pulse Streamer out"=w238:refnum<class "PulseStreamer.lvclass">)  [unwired: 8 in]
                n52 = call <vilib>:"Add Level.vi"("Level"=FALSE, "Duration"=w189, "Digital Sequence in"=w217) -> ("Digital Sequence out"=w215:refnum<class "PulsePattern.lvclass">)  [unwired: 8 in]
                n53 = call-dynamic "createSequence.vi"("error in (no error)"=w239, "PulseStreamer in"=w238) -> ("error out"=w187:errorcluster, "Sequence"=w188:refnum<class "Sequence.lvclass">, "PulseStreamer out"=w226:refnum<class "PulseStreamer.lvclass">)  [unwired: 7 in]
                n54 = call <vilib>:"Add Level.vi"("Level"=TRUE, "Duration"=w195, "Digital Sequence in"=refnum<class "PulsePattern.lvclass"> refnum) -> ("Digital Sequence out"=w233:refnum<class "PulsePattern.lvclass">)  [unwired: 8 in]
                n55 = call <vilib>:"Add Level.vi"("Level"=TRUE, "Duration"=i64 100, "Digital Sequence in"=refnum<class "PulsePattern.lvclass"> refnum) -> ("Digital Sequence out"=w179:refnum<class "PulsePattern.lvclass">)  [unwired: 8 in]
                n56 = call <vilib>:"Add Level.vi"("Level"=TRUE, "Duration"=i64 100, "Digital Sequence in"=refnum<class "PulsePattern.lvclass"> refnum) -> ("Digital Sequence out"=w167:refnum<class "PulsePattern.lvclass">)  [unwired: 8 in]
                n57 = call <vilib>:"Add Level.vi"("Level"=FALSE, "Duration"=w190, "Digital Sequence in"=w215) -> ("Digital Sequence out"=w248:refnum<class "PulsePattern.lvclass">)  [unwired: 8 in]
                n58 = call <vilib>:"Add Level.vi"("Level"=FALSE, "Duration"=w190, "Digital Sequence in"=w233) -> ("Digital Sequence out"=w232:refnum<class "PulsePattern.lvclass">)  [unwired: 8 in]
                n59 = Add(x=w218, y=w189) -> (x+y=w194:T1)
                n60 = call <vilib>:"Add Level.vi"("Level"=TRUE, "Duration"=w189, "Digital Sequence in"=w248) -> ("Digital Sequence out"=w186:refnum<class "PulsePattern.lvclass">)  [unwired: 8 in]
                n61 = call <vilib>:"Add Level.vi"("Level"=TRUE, "Duration"=w194, "Digital Sequence in"=w232) -> ("Digital Sequence out"=w185:refnum<class "PulsePattern.lvclass">)  [unwired: 8 in]
                n62 = call <vilib>:"Add Level.vi"("Level"=w203, "Duration"=w202, "Digital Sequence in"=w186) -> ("Digital Sequence out"=w207:refnum<class "PulsePattern.lvclass">)  [unwired: 8 in]
                n63 = call <vilib>:"Add Level.vi"("Level"=TRUE, "Duration"=w195, "Digital Sequence in"=w185) -> ("Digital Sequence out"=w200:refnum<class "PulsePattern.lvclass">)  [unwired: 8 in]
                n64 = call <vilib>:"Add Level.vi"("Level"=w203, "Duration"=w189, "Digital Sequence in"=w207) -> ("Digital Sequence out"=w206:refnum<class "PulsePattern.lvclass">)  [unwired: 8 in]
                n65 = call <vilib>:"Add Level.vi"("Level"=FALSE, "Duration"=w190, "Digital Sequence in"=w200) -> ("Digital Sequence out"=w199:refnum<class "PulsePattern.lvclass">)  [unwired: 8 in]
                n66 = call <vilib>:"Add Level.vi"("Level"=w203, "Duration"=w190, "Digital Sequence in"=w206) -> ("Digital Sequence out"=w205:refnum<class "PulsePattern.lvclass">)  [unwired: 8 in]
                n67 = call <vilib>:"Add Level.vi"("Level"=TRUE, "Duration"=i64 100, "Digital Sequence in"=w167) -> ("Digital Sequence out"=w166:refnum<class "PulsePattern.lvclass">)  [unwired: 8 in]
                n68 = call <vilib>:"Add Level.vi"("Level"=TRUE, "Duration"=w189, "Digital Sequence in"=w205) -> ("Digital Sequence out"=w204:refnum<class "PulsePattern.lvclass">)  [unwired: 8 in]
                n69 = call-dynamic "setDigital.vi"("error in (no error)"=w187, "PulsePattern"=w204, "channel"=T3 2, "Sequence in"=w188) -> ("error out"=w234:errorcluster, "Sequence out"=w235:refnum<class "Sequence.lvclass">)  [unwired: 6 in]
                n70 = call <vilib>:"Add Level.vi"("Level"=TRUE, "Duration"=w194, "Digital Sequence in"=w199) -> ("Digital Sequence out"=w198:refnum<class "PulsePattern.lvclass">)  [unwired: 8 in]
                n71 = call <vilib>:"Add Level.vi"("Level"=FALSE, "Duration"=i64 500, "Digital Sequence in"=w179) -> ("Digital Sequence out"=w192:refnum<class "PulsePattern.lvclass">)  [unwired: 8 in]
                n72 = call-dynamic "setDigital.vi"("error in (no error)"=w234, "PulsePattern"=w198, "channel"=T3 0, "Sequence in"=w235) -> ("error out"=w210:errorcluster, "Sequence out"=w209:refnum<class "Sequence.lvclass">)  [unwired: 6 in]
                n73 = call-dynamic "setDigital.vi"("error in (no error)"=w210, "PulsePattern"=w192, "channel"=T3 3, "Sequence in"=w209) -> ("error out"=w171:errorcluster, "Sequence out"=w173:refnum<class "Sequence.lvclass">)  [unwired: 6 in]
                n74 = call-dynamic "setDigital.vi"("error in (no error)"=w171, "PulsePattern"=w166, "channel"=T3 1, "Sequence in"=w173) -> ("error out"=w170:errorcluster, "Sequence out"=w172:refnum<class "Sequence.lvclass">)  [unwired: 6 in]
                n75 = call <vilib>:"repeat.vi"("error in (no error)"=w170, "Repeat count"=w181, "Sequence in"=w172) -> ("error out"=w184:errorcluster, "Sequence out"=w183:refnum<class "Sequence.lvclass">)  [unwired: 7 in]
                n76 = call <vilib>:"getDuration.vi"("Sequence in"=w183) -> ("Sequence duration [ns]"=w182:i64, "Sequence out"=w244:refnum<class "Sequence.lvclass">)  [unwired: 9 in]
                n77 = Divide(x=w182, y=i64 1000000) -> (x/y=w161:dbl)
                "64bit integer" <- w161
                n78 = call <vilib>:"plot.vi"("Sequence in"=w244) -> ("Digital plot"=→"Digital plot":cluster{"CumTime":i64[], dbl[]}[], "Sequence out"=w225:refnum<class "Sequence.lvclass">)  [unwired: 7 in, 2 out]
                n79 = local read "Pulse Num"() -> (w180:u32)
                n80 = call-dynamic "setTrigger.vi"("error in (no error)"=w184, "start"="start", "Pulse Streamer in"=w226) -> ("error out"=w228:errorcluster, "Pulse Streamer out"=w227:refnum<class "PulseStreamer.lvclass">)  [unwired: 7 in]
                n81 = Divide(x=w182, y=w181) -> (x/y=w176:dbl)
                n82 = Divide(x=w176, y=2.0) -> (x/y=→"t_tot single sequence (ns)":dbl)
                n83 = To Quad Integer(1:w180) -> (0:w220:i64)
                "n_runs" <- w220
                n84 = Multiply(x=w220, y=w161) -> (x*y=→"Sequence duration [ms]":dbl)
                n85 = call-poly <vilib>:"stream.vi"("error in (no error)"=w228, "n_runs"=w220, "sequence"=w225, "Pulse Streamer in"=w227) -> ("error out"=→"error out 3":errorcluster)  [unwired: 4 in, 1 out]
              }
              frame #2 {
                n86 = local read "Number of points"() -> (w252:u32)
                n87 = local read "Pulse Num"() -> (w256:u32)
                n88 = Multiply(x=u32 2 ("y"), y=w252) -> (x*y=w250:u32)
                n89 = Multiply(x=w256, y=w250) -> (x*y=w255:u32)
                n90 = local read "Number of points"() -> (w254:u32)
                n91 = xnode "Invoke Method"("FPGA VI Reference In"=w260, "error in"=w259, "Number of Elements"=w255, "Timeout (ms)"=-1) -> ("FPGA VI Reference Out"=w258:refnum<k20>, "error out"=w257:errorcluster, "Data"=w261:u32[], "Elements Remaining"=→"Elements Remaining":u32)
                n92 = local read "Pulse Num"() -> (w253:u32)
              }
              frame #3 {
                w266 = u32[] []
                w277 = 2 ("dimension size")
                # "readout"
                # "Initial"
                n93 = Array Size(array=w279) -> (size(s)=w278:i32)
                n94 = Divide(x=w278, y=w277) -> (x/y=w269:dbl)
                n95 = Reshape Array(w279, w269, w277) -> (w276:u32[][])
                n96 = Index Array(array=w276, index (col) #1=0 ("disabled index (col)"), index (col) #2=1 ("disabled index (col)")) -> (element #1=w273:u32[], element #2=w272:u32[])  [unwired: 2 in]
                n97 = Add Array Elements(numeric array=w273) -> (sum=w285:u32)
                n98 = Reshape Array(w272, w271, w270) -> (w282:u32[][])
                n99 = Reshape Array(w273, w271, w270) -> (w284:u32[][])
                n100 = Transpose 2D Array(2D array=w282) -> (transposed array=w281:u32[][])
                n101 = Transpose 2D Array(2D array=w284) -> (transposed array=w283:u32[][])
                n102 = for {
                  N: w270 -> [_]
                  tunnel: w281 -> [w296] mode=indexing
                  shift-right: [w295] -> w280
                  shift-left: dbl[] [] -> [w292]
                  tunnel: w283 -> [w293] mode=indexing
                  shift-right: [w289] -> w265
                  shift-left: w266 -> [w290]
                  shift-right: [w286] -> w264
                  shift-left: w266 -> [w287]
                  n103 = Add Array Elements(numeric array=w296) -> (sum=w288:u32)
                  n104 = Add Array Elements(numeric array=w293) -> (sum=w291:u32)
                  n105 = Insert Into Array(array=w290, new element=w291) -> (w289:u32[])  [unwired: 1 in]
                  n106 = Insert Into Array(array=w287, new element=w288) -> (w286:u32[])  [unwired: 1 in]
                  n107 = Divide(x=w291, y=w288) -> (x/y=w294:dbl)
                  n108 = Insert Into Array(array=w292, new element=w294) -> (w295:dbl[])  [unwired: 1 in]
                }
                n109 = local read "Experiment number"() -> (w268:i32)
              }
            }
            n110 = To Double Precision Float(number=w87) -> (double precision float=w86:dbl[])
            n111 = To Double Precision Float(number=w84) -> (double precision float=w83:dbl[])
            n112 = local read "tau array"() -> (w82:dbl[])
            n113 = xnode "Close FPGA VI Reference"("FPGA VI Reference In"=w107, "error in"=w106) -> ("error out"=→"error out 4":errorcluster)
            n114 = Not Equal?(x=0, y=w85) -> (x != y?=w77:bool)
            n115 = case shown="True" w77 {
              tunnel: [w126 w133] -> w80
              tunnel: w86 -> [w126 w127]
              tunnel: w85 -> [_ w128]
              frame False {
              }
              frame True {
                n116 = local read "Ave F1"() -> (w132:dbl[])
                n117 = Multiply(x=w132, y=w128) -> (x*y=w131:dbl[])
                n118 = Add(x=w127, y=w131) -> (x+y=w130:dbl[])
                n119 = Increment(x=w128) -> (x+1=w129:i32)
                n120 = Divide(x=w130, y=w129) -> (x/y=w133:dbl[])
              }
            }
            n121 = case shown="True" w77 {
              tunnel: [w118 w125] -> w81
              tunnel: w83 -> [w118 w119]
              tunnel: w85 -> [_ w120]
              frame False {
              }
              frame True {
                n122 = local read "Ave F2"() -> (w124:dbl[])
                n123 = Multiply(x=w124, y=w120) -> (x*y=w123:dbl[])
                n124 = Add(x=w119, y=w123) -> (x+y=w122:dbl[])
                n125 = Increment(x=w120) -> (x+1=w121:i32)
                n126 = Divide(x=w122, y=w121) -> (x/y=w125:dbl[])
              }
            }
            n127 = case shown="False" w77 {
              tunnel: [w297 w304] -> w116
              tunnel: w92 -> [w297 w303]
              tunnel: w85 -> [_ w298]
              frame False {
              }
              frame True {
                n128 = local read "Averaged ESR"() -> (w302:dbl[])
                n129 = Multiply(x=w302, y=w298) -> (x*y=w301:dbl[])
                n130 = Add(x=w303, y=w301) -> (x+y=w300:dbl[])
                n131 = Increment(x=w298) -> (x+1=w299:i32)
                n132 = Divide(x=w300, y=w299) -> (x/y=w304:dbl[])
              }
            }
            n133 = local read "CountAverage"() -> (w115:dbl[])
            n134 = Bundle("tau array"=w82, w80) -> (→"ESR F1":cluster{"tau array":dbl[], dbl[]})  [unwired: 1 in]
            n135 = Bundle("tau array"=w82, w81) -> (→"ESR F2":cluster{"tau array":dbl[], dbl[]})  [unwired: 1 in]
            n136 = Divide(x=w89, y=w88) -> (x/y=w105:dbl)
            n137 = Insert Into Array(array=w115, new element=w105) -> (w114:dbl[])  [unwired: 1 in]
            n138 = Bundle("tau array"=w82, w116) -> (→"Rabi plot":cluster{"tau array":dbl[], dbl[]})  [unwired: 1 in]
            n139 = local read "N_array"() -> (w113:i32[])
            n140 = Bundle("N_array"=w113, "CountAverage"=w114) -> (→"Average Counts":cluster{"N_array":i32[], "CountAverage":dbl[]})  [unwired: 1 in]
          }
        }
        "Ave F1" <- w22
        "Ave F2" <- w21
      }
    }
  }
